vi "FixPixmap.vi"(8 "error in (no error)":errorcluster, 11 "image data in":T1) -> (0 "error out":errorcluster, 3 "image data out":T1)   [LabVIEW 2020, in "g_ar_toolkit.image.lvlib"]
uses:
  g_ar_toolkit.image.lvlib
  <vilib>/picture/picture.llb/imagedata.ctl
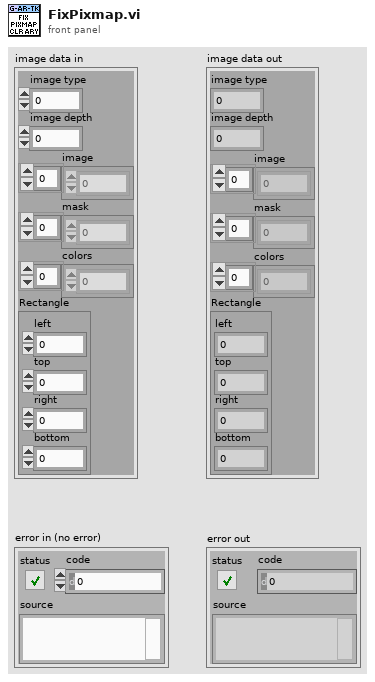
[diagram p1: front panel]
types:
  T1 = typedef "imagedata.ctl" = cluster{"image type":i32, "image depth":i32, "image":u8[], "mask":u8[], "colors":u32[], "Rectangle":cluster{"left":i16, "top":i16, "right":i16, "bottom":i16}}
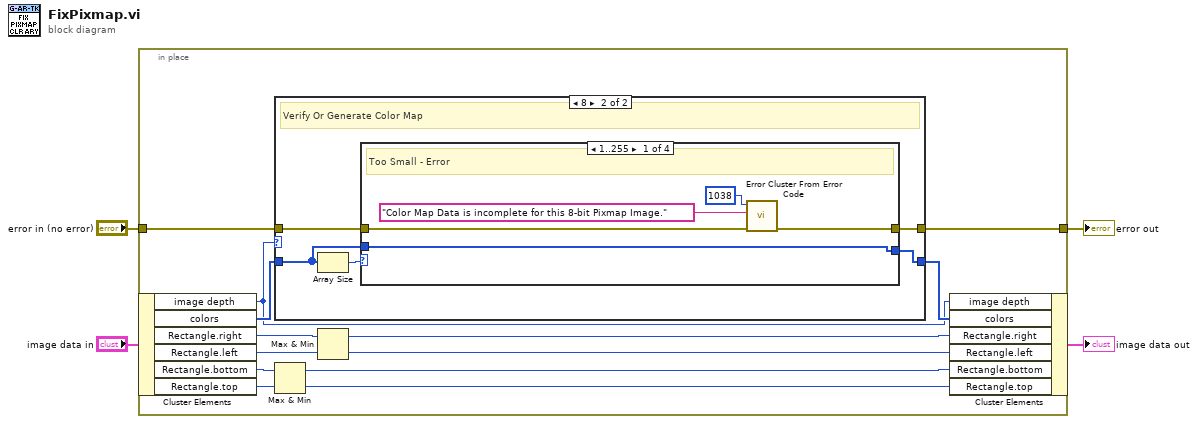
[diagram p0: block diagram]
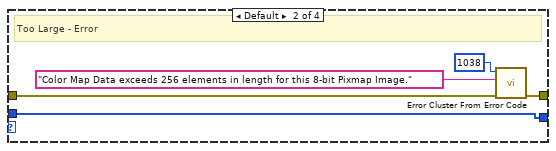
[diagram p3: hidden frame]
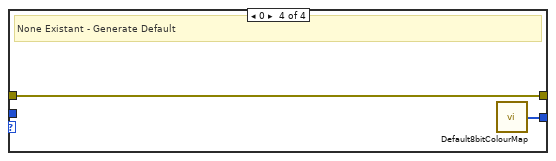
[diagram p5: hidden frame]
diagram:
  n1 = in-place {
    in-place-border: "error in (no error)" -> [w14]
    in-place-border: [w13] -> w1
    n2 = in-place-cluster #1("image data in") -> ("image depth"=w15:i32, "colors"=w17:u32[], "Rectangle.right"=w12:i16, "Rectangle.left"=w11:i16, "Rectangle.bottom"=w8:i16, "Rectangle.top"=w5:i16)
    n3 = case shown="8" w15 {
      tunnel: w17 -> [w19 w22]
      tunnel: [w19 w23] -> w16
      tunnel: w14 -> [w18 w21]
      tunnel: [w18 w20] -> w13
      frame Default {
        # "No Colors Array to Worry About"
      }
      frame 8 {
        # "Verify Or Generate Color Map"
        n4 = Array Size(array=w22) -> (size(s)=w24:i32)
        n5 = case shown="1..255" w24 {
          tunnel: [w29 w34 w36 w38] -> w23
          tunnel: w22 -> [w29 w34 w36 _]
          tunnel: w21 -> [w28 w33 w35 w37]
          tunnel: [w25 w30 w35 w37] -> w20
          frame 1..255 {
            # "Too Small - Error"
            n6 = call <vilib>:"Error Cluster From Error Code.vi"("error in (no error)"=w28, "error message (\"\")"="Color Map Data is incomplete for this 8-bit Pixmap Image." ("error message (\"\")"), "error code (0)"=1038) -> ("error out"=w25:errorcluster)  [unwired: 6 in]
          }
          frame Default {
            # "Too Large - Error"
            n7 = call <vilib>:"Error Cluster From Error Code.vi"("error in (no error)"=w33, "error message (\"\")"="Color Map Data exceeds 256 elements in length for this 8-bit Pixmap Image." ("error message (\"\")"), "error code (0)"=1038) -> ("error out"=w30:errorcluster)  [unwired: 6 in]
          }
          frame 256 {
            # "Just Right - Pass Through"
          }
          frame 0 {
            # "None Existant - Generate Default"
            n8 = call "Default8bitColourMap.vi"() -> ("Default 8-bit Colour Map"=w38:u32[])
          }
        }
      }
    }
    n9 = Max & Min(x=w8, y=w5) -> (max(x,y)=w7:i16, min(x,y)=w6:i16)
    n10 = Max & Min(x=w12, y=w11) -> (max(x,y)=w10:i16, min(x,y)=w9:i16)
    n11 = in-place-cluster #1("image depth"=w15, "colors"=w16, "Rectangle.right"=w10, "Rectangle.left"=w9, "Rectangle.bottom"=w7, "Rectangle.top"=w6) -> (→"image data out":T1)
  }
  "error out" <- w1
